vi "prueba sonido nueva.vi"() -> ()   [LabVIEW 2010]
uses:
  <vilib>/sound2/lvsound2.llb/Sound Data Format.ctl
  <vilib>/sound2/lvsound2.llb/Sound Output Task ID.ctl
panel:
  in  "Frecuencia":dbl
  in  "stop":bool
  out "Waveform":waveform(dbl)(graph)
  in  "Sound?":bool
  in  "Sound Controls":T2={"device ID"=0, "sound format"={"sample rate (S/s)"=44000.0, "number of channels"=2, "bits per sample"=16}, "time (ms)"=200.0}
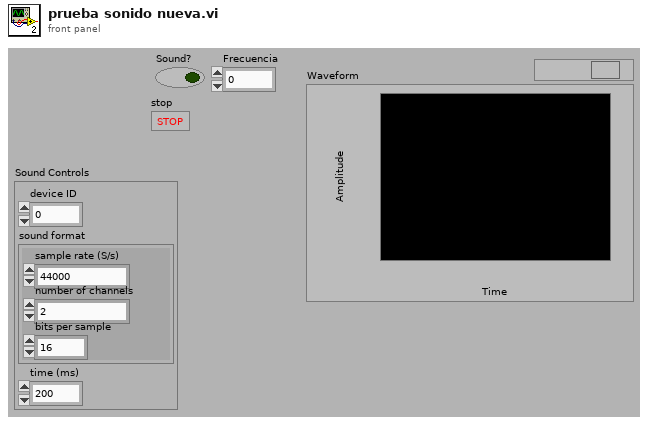
[diagram p1: front panel]
types:
  T1 = typedef "Sound Data Format.ctl" = cluster{"sample rate (S/s)":dbl, "number of channels":i32, "bits per sample":i32}
  T2 = cluster{"device ID":u32, "sound format":T1, "time (ms)":dbl}
  T3 = typedef "Sound Output Task ID.ctl" = u32
  T4 = cluster{"task ID":T3, "error":errorcluster, "sound format":T1}
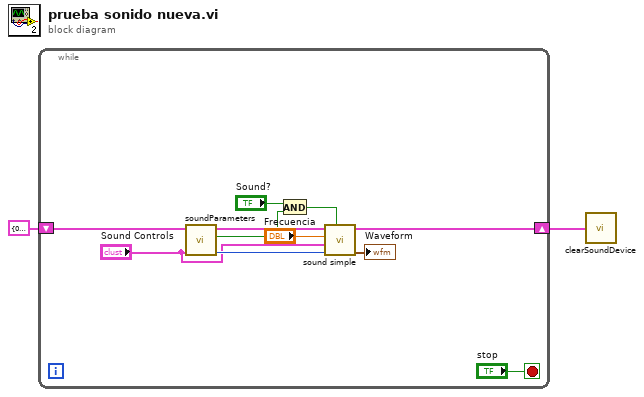
[diagram p0: block diagram]
diagram:
  n1 = while {
    shift-right: [w10] -> w2
    shift-left: T4 {"task ID"=0, "error"={"status"=TRUE, "code"=0, "source"=""}, "sound format"={"sample rate (S/s)"=0.0, "number of channels"=0, "bits per sample"=0}} ("Sound Device OUT") -> [w11]
    stop <- "stop" stop-if-true
    n2 = call "soundParameters.vi"("Sound Controls"="Sound Controls", "Sound Device IN"=w11) -> ("#samples"=w13:u32, "En funcionamiento?"=w7:bool, "Sound Device OUT"=w12:T4)  [unwired: 3 in]
    n3 = And(x="Sound?", y=w7) -> (x .and. y?=w8:bool)
    n4 = call "sound simple.vi"("sound?"=w8, "# samples"=w13, "Sound Parameters"="Sound Controls", "Frecuencia"="Frecuencia", "Sound Device IN"=w12) -> ("Waveform"=→"Waveform":waveform(dbl), "Sound Device OUT"=w10:T4)  [unwired: 3 in]
  }
  n5 = call "clearSoundDevice.vi"("Sound Device OUT"=w2) -> ()
